vi "MB_string_generator_preliminary.vi"() -> ()   [LabVIEW 2019]
panel:
  in  "Number of bits to read(4 digits)":string="\u0000\u0002"
  out "String out":string
  in  "Register number":u16=18735
  in  "Function in hex":string="\u0003"
  in  "Drive address in hex":string="\u0002"
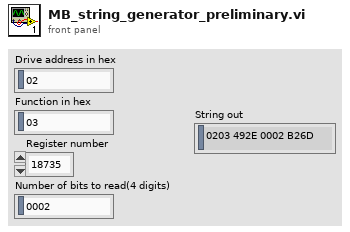
[diagram p1: front panel]
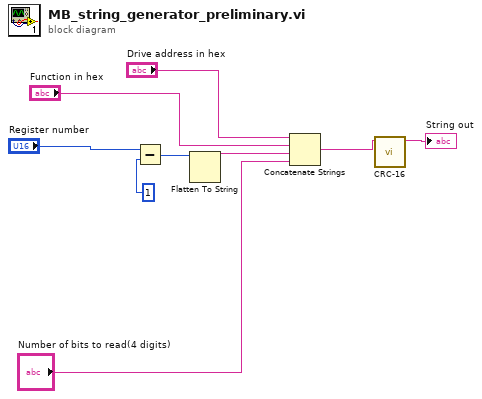
[diagram p0: block diagram]
diagram:
  n1 = Subtract(x="Register number", y=u16 1) -> (x-y=w4:u16)
  n2 = Flatten To String(anything=w4) -> (data string=w3:string)  [unwired: 3 in, 2 out]
  n3 = Concatenate Strings("Drive address in hex", "Function in hex", w3, "Number of bits to read(4 digits)") -> (w2:string)
  n4 = call "CRC-16.vi"("String in"=w2) -> ("String out"=→"String out":string)  [unwired: 8 in, 2 out]
